vi "File Append.vi"(1 "function (open:0)":T1(ring)=enum."open or create", 2 "string":string, 3 "file path":path) -> ()   [LabVIEW 2017]
panel:
  out "error out":errorcluster
  out "path":path
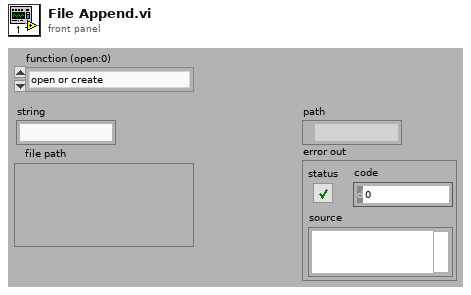
[diagram p1: front panel]
types:
  T1 = enum16{"open", "open or create", "create or replace", "create", "open (read only)"}
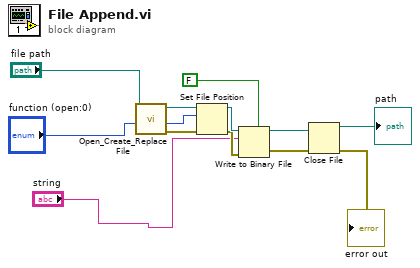
[diagram p0: block diagram]
diagram:
  n1 = call <vilib>:"Open_Create_Replace File.vi"("function (open:0)"="function (open:0)", "file path"="file path") -> ("error out"=w12:errorcluster, "file size (bytes)"=w10:i32, "refnum"=w11:refnum<file>)  [unwired: 6 in, 1 out]
  n2 = Set File Position(offset (in bytes) (0)=w10, refnum=w11, error in=w12) -> (refnum out=w7:refnum<file>, error out=w6:errorcluster)  [unwired: 1 in]
  n3 = Write to Binary File(file (use dialog)=w7, data="string", error in=w6, 5:FALSE ("prepend array or string size? (T)")) -> (refnum out=w8:refnum<file>, error out=w9:errorcluster)  [unwired: 2 in, 1 out]
  n4 = Close File(refnum=w8, error in=w9) -> (path=→"path":path, error out=→"error out":errorcluster)
